vi "CONEX-LDS Set Units Coefficient v2.vi"(9 "Units Coefficient":string, 11 "Connection Cluster in":T1) -> (3 "Connection Cluster out":T1)   [LabVIEW 2010]
doc: "SU - Set Units Coefficient\n\nInput: New Units Coefficient {string} value\n\nUnits can be up to 5 characters long and should be set to match calibration values set with PX and PY. The string set is only for informative reasons, as user has complete control of calibration values. To return to factory settings: Query CD to get factory settings and use PX, PY and SU to set back to factory settings."
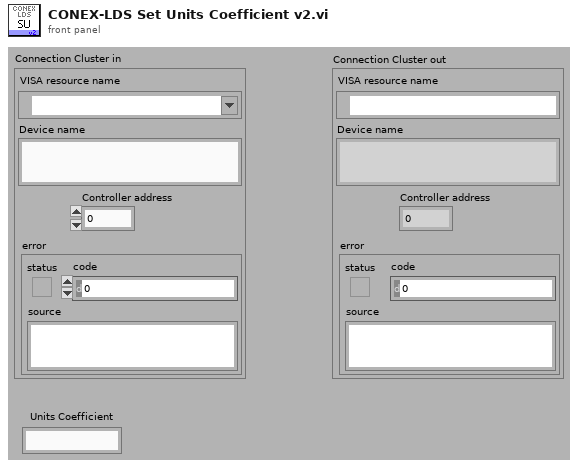
[diagram p1: front panel]
types:
  T1 = cluster{"VISA resource name":refnum<visa-resource-name>, "Device name":string, "Controller address":i32, "error":errorcluster}
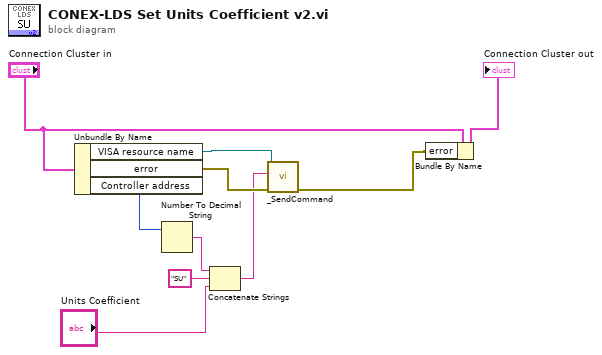
[diagram p0: block diagram]
diagram:
  n1 = Unbundle By Name("Connection Cluster in") -> ("VISA resource name"=w8:refnum<visa-resource-name>, "error"=w6:errorcluster, "Controller address"=w3:i32)
  n2 = Number To Decimal String(number=w3) -> (decimal integer string=w10:string)  [unwired: 1 out]
  n3 = Concatenate Strings(w10, "SU" ("strCommand"), "Units Coefficient") -> (w2:string)
  n4 = call <userlib>:"_SendCommand.vi"("error in"=w6, "Command"=w2, "Instrument Channel"=w8) -> ("error out"=w7:errorcluster)  [unwired: 7 in, 1 out]
  n5 = Bundle By Name(cluster="Connection Cluster in", "error"=w7) -> (→"Connection Cluster out":T1)
